vi "Get Set Create Sensor Key Focus.vi"(8 "error in (no error)":errorcluster, 11 "Abstract Set Create Sensor Key Focus Msg in":refnum<class "Abstract Set Create Sensor Key Focus Msg.lvclass">) -> (0 "error out":errorcluster, 2 "Set Create Sensor Key Focus":bool, 3 "Abstract Set Create Sensor Key Focus Msg out":refnum<class "Abstract Set Create Sensor Key Focus Msg.lvclass">)   [LabVIEW 2013, in "Create Sensor Model.lvlib" / "Abstract Set Create Sensor Key Focus Msg.lvclass"]
uses:
  Abstract Set Create Sensor Key Focus Msg.lvclass
  Abstract Set Create Sensor Key Focus Msg.lvclass/Abstract Set Create Sensor Key Focus Msg.ctl
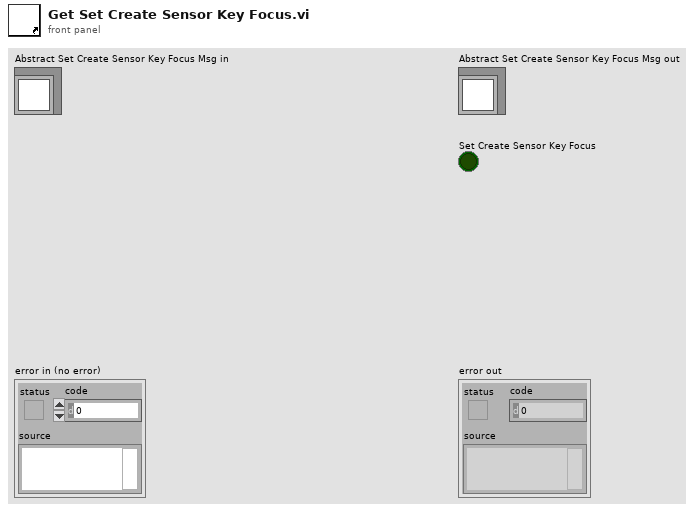
[diagram p1: front panel]
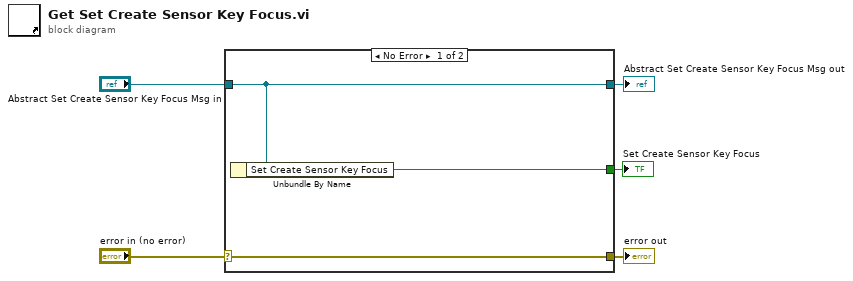
[diagram p0: block diagram]
diagram:
  n1 = case shown="No Error" "error in (no error)" {
    selector: "error in (no error)" -> [w8 w9]
    tunnel: [w8 w9] -> w4
    tunnel: [w7 w10] -> w2
    tunnel: "Abstract Set Create Sensor Key Focus Msg in" -> [w7 w10]
    tunnel: [w6 _] -> w1
    frame No Error {
      n2 = Unbundle By Name(w7) -> ("Set Create Sensor Key Focus"=w6:bool)
    }
    frame Error {
    }
  }
  "error out" <- w4
  "Abstract Set Create Sensor Key Focus Msg out" <- w2
  "Set Create Sensor Key Focus" <- w1
